vi "Udp Tester 4.vi"() -> ()   [LabVIEW 2014]
uses:
  <vilib>/addons/control/pid/pid.llb/PID (DBL).vi
  <vilib>/addons/control/pid/pid.llb/PID Percentage to EGU (DBL).vi
  <vilib>/FPGAPlugInAG/myRIO-1900/niLvFpga_Open_myRIO-1900.vi
  <vilib>/rvi/interface/common/dynamic/niFpgaDynamicAddResources.vi
  <vilib>/Utility/error.llb/Error Cluster From Error Code.vi
  <vilib>/rvi/errors/niLvFpgaAdjustHostInterfaceError.vi
  <vilib>/FPGAPlugInAG/Dynamic/niLvFpga_Close_Dynamic.vi
  <vilib>/rvi/interface/nirviOpenFPGA/nirviOpenFPGA.xnode
  FPGA Bitfiles/Test_FPGATarget_CurrentControl_60eBuCSPTsI.lvbitx
  Current Control.vi
  <vilib>/rvi/interface/nirviReadWriteControl/nirviReadWriteControl.xnode
  <vilib>/rvi/interface/nirviCloseFPGA/nirviCloseFPGA.xnode
  <vilib>/addons/control/pid/NI_PID_pid.lvlib
  NiFpgaLv.dll
  <vilib>/rvi/interface/Simulation/niFpgaSimulationCallBeginRW.vi
  <vilib>/Utility/file.llb/Write To Spreadsheet File (I64).vi
panel:
  out "Status?":bool
  in  "Tab Control 2":T1(tab)
  out "Plant Output vs. IAB Height":waveform(dbl)[](graph)=[{"t0"=timestamp(1835.8000000000002 s since 1904-01-01), "dt"=1.0, "Y"=[0.9645428084016676]}, {"t0"=timestamp(1835.8000000000002 s since 1904-01-01), "dt"=1.0, "Y"=[1.0]}]
  in  "SP1: 2":dbl(slide)=40.87020302841148 min=0.0 max=0.0 scale=35.0..43.0
  out "Head Pose:":dbl(slide)=50.762476114859936 scale=0.0..100.0
  out "Static Response":cluster{dbl, "Input Signal":dbl}[](graph)
  out "Excitation":cluster{"Time":dbl[], "Signal":dbl[]}(graph)
  out "Response":cluster{"Time":dbl[], "Signal":dbl[]}(graph)
  in  "stop":bool
  out "SP and PV":cluster{"Plant Output":dbl, "SP:":dbl}(graph)
  out "MV (mA)":dbl(graph)=20.39115328927357
  in  "Loop Cycle":i32
  in  "Tab Control":enum32{"Profile", "Diagram"}(tab)
  out "Inflow Profile Graph":cluster{dbl, dbl}[](graph)
  in  "Apply Inflow Profile":bool=TRUE
  in  "Constant Flow (%)":dbl=40.0
  in  "Inflow Profile":cluster{"time (s)":dbl, "setpoint":dbl}[](array[cluster])=[{"time (s)"=0.0, "setpoint"=40.0}, {"time (s)"=10.0, "setpoint"=40.0}, {"time (s)"=10.0, "setpoint"=60.0}, {"time (s)"=20.0, "setpoint"=60.0}]
  out "FT Valve":dbl(knob)=84.28886007445381 scale=0.0..190.0
  out "control valve":dbl=86.66603993277398 format="%.2f"
  out "Valve":bool
  out "Pump":bool=TRUE
  out "Bladder Tank":dbl(slide)=49.279730305904245 scale=0.0..100.0 scale format="%.2f"
  out "FT":dbl(knob)=84.28886007445381 scale=0.0..100.0
  out "PV 1":dbl=49.279730305904245
  in  "Stop":bool
  in  "PID parameters (LC)":T2={"Kc"=-20.0, "Ti (min)"=0.1, "Td (min)"=0.0} {"Td (min)" format="%#.6f"; "Ti (min)" format="%#.4f"; "Kc" format="%#.4f"}
  in  "SP1:":dbl(slide)=40.87020302841148 min=0.0 max=0.0 scale=0.0..100.0
  out "PV1:":dbl(slide)=50.762476114859936 scale=0.0..190.0
  out "MV1:":dbl(slide)=100.0 scale=-100.0..100.0
  # "Time (s)"
  # "Flow (%)"
  # "SP"
  # "///"
  # "///"
  # "///"
  # "1"
  # "///"
  # "SP"
  # "2"
  # "mA"
  # "mA"
  # "FC"
  # "LT"
  # "1"
  # "+"
  # "+"
  # "S"
  # "LC"
  # "FT"
  # "1"
  # "%"
  # "cm"
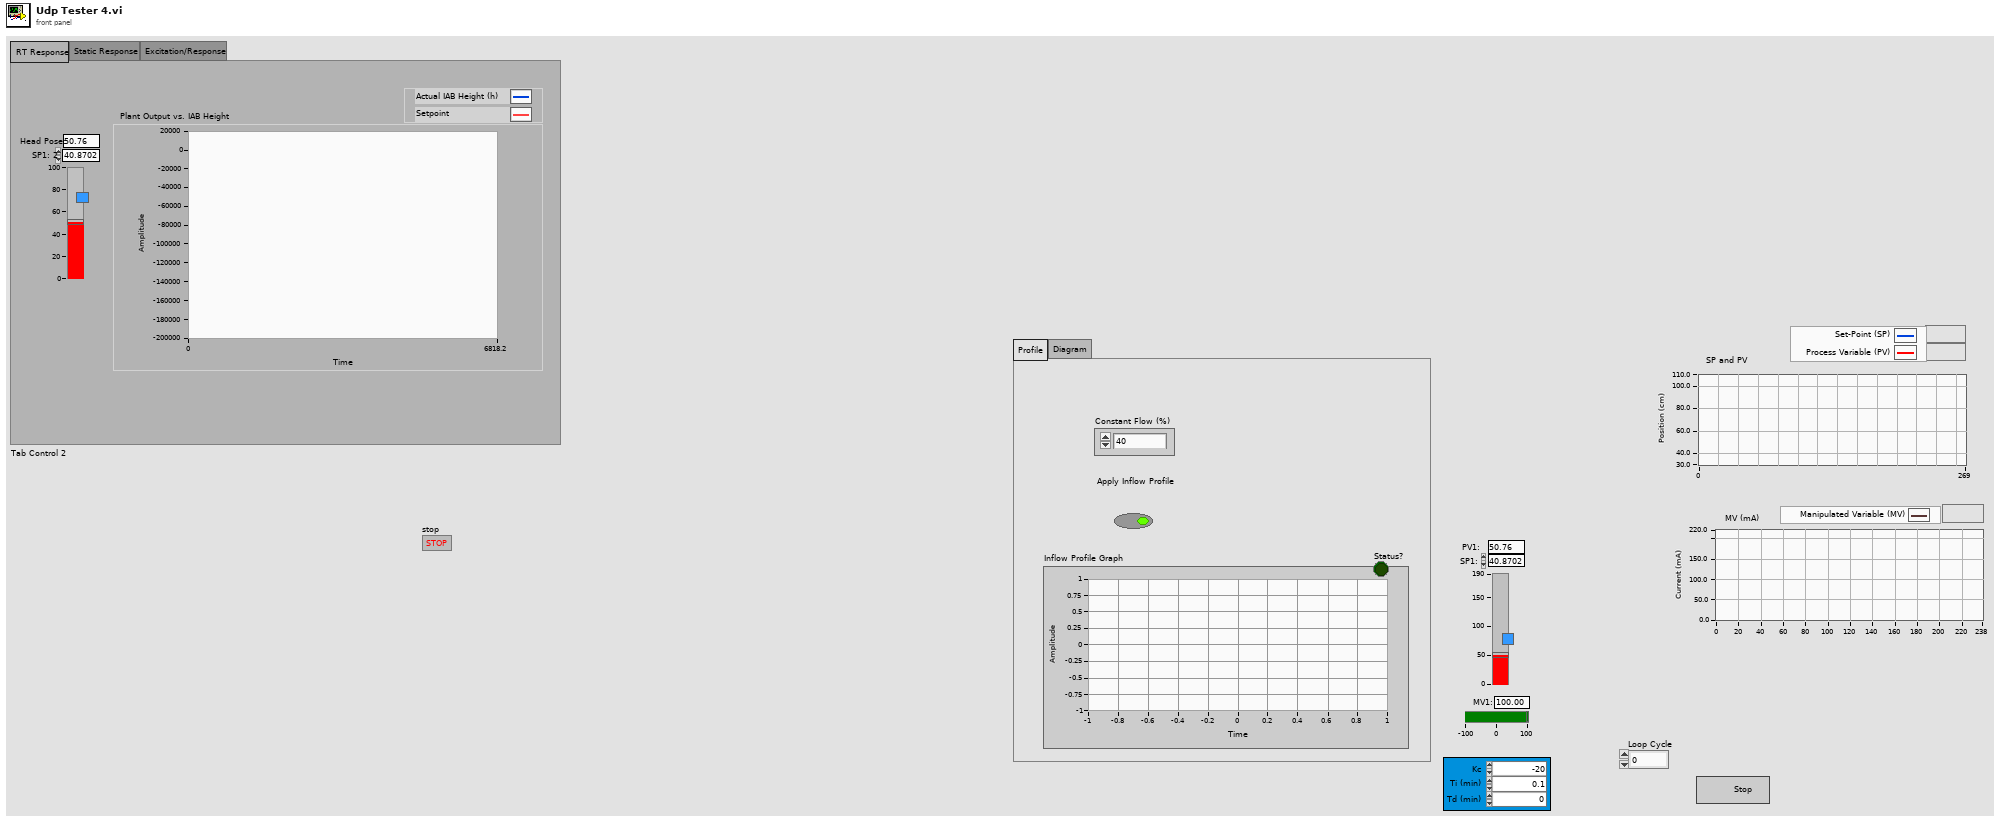
[diagram p1: front panel]
types:
  T1 = enum32{"RT Response", "Static Response", "Excitation/Response"}
  T2 = cluster{"Kc":dbl, "Ti (min)":dbl, "Td (min)":dbl}
  T3 = enum16{"big-endian, network order", "native, host order", "little-endian"}
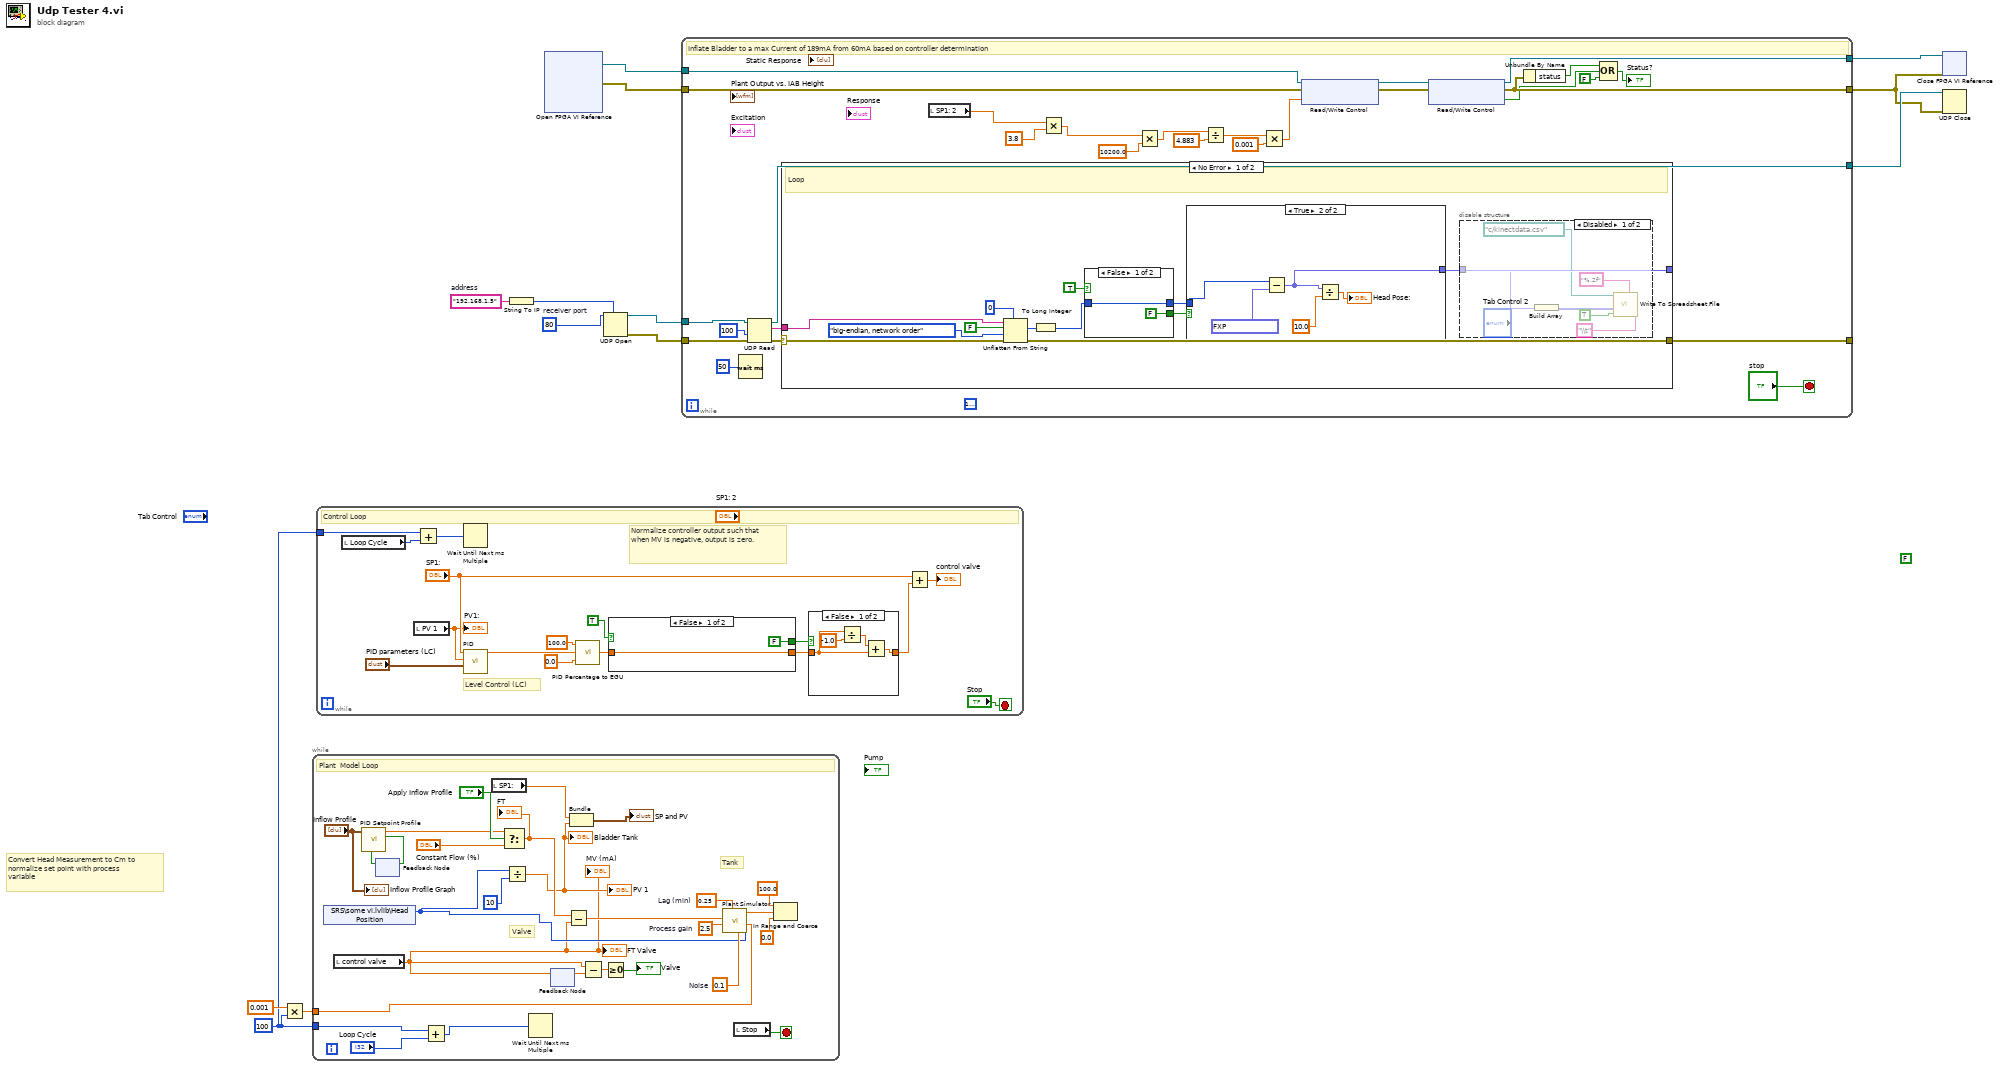
[diagram p0: block diagram]
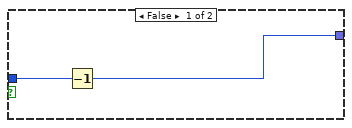
[diagram p3: hidden frame]
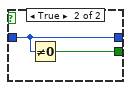
[diagram p4: hidden frame]
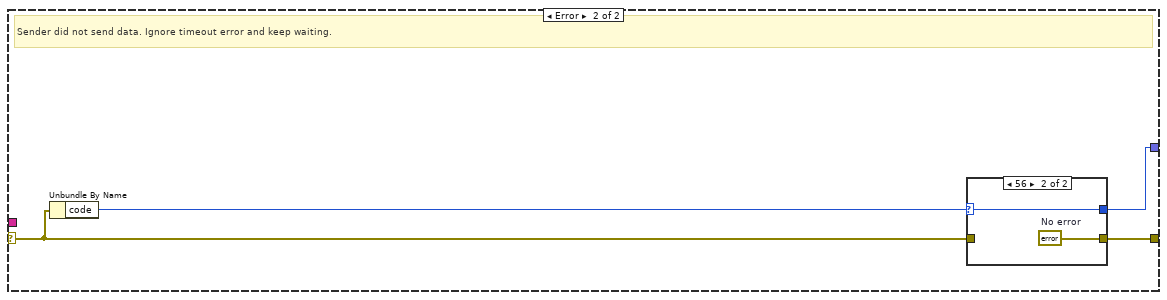
[diagram p5: hidden frame]
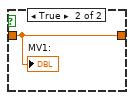
[diagram p7: hidden frame]
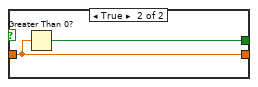
[diagram p8: hidden frame]
diagram:
  w9 = "192.168.1.5"  # address
  w8 = u16 80  # receiver port
  w11 = 100
  (unwired) FALSE
  # "Convert Head Measurement to Cm to normalize set point with process variable"
  n1 = Multiply(x=0.001, y=w11) -> (x*y=w12:dbl)
  n2 = while {
    tunnel: w12 -> [w27]
    tunnel: w11 -> [w18]
    stop <- w39 stop-if-true
    w37 = 0.25  # Lag (min)
    w36 = 2.5  # Process gain
    w35 = 0.1  # Noise
    # "Tank"
    # "Valve"
    # "Plant  Model Loop"
    n3 = shared-variable "SRS\\some vi.lvlib\\Head Position"() -> (w21:i32)  [unwired: 1 in, 1 out]
    n4 = local read "control valve"() -> (w16:dbl)
    "FT Valve" <- w16
    "MV (mA)" <- w16
    n5 = feedback #1() -> (w40:bool)  [unwired: 1 in]
    n6 = call <vilib>:"PID Setpoint Profile.vi"("reinitialize? (F)"=w40, "setpoint profile"="Inflow Profile") -> ("profile complete?"=w41:bool, "setpoint"=w29:dbl)  [unwired: 4 in, 2 out]
    n7 = feedback-in #1(w41) -> ()
    n8 = Add(x=w18, y="Loop Cycle") -> (x+y=w19:i32)
    n9 = local read "SP1:"() -> (w15:dbl)
    n10 = Select(t=w29, s="Apply Inflow Profile", f="Constant Flow (%)") -> (s? t:f=w30:dbl)
    "FT" <- w30
    n11 = Divide(x=w21, y=10 ("x")) -> (x/y=w22:dbl)
    "Bladder Tank" <- w22
    "PV 1" <- w22
    n12 = Wait Until Next ms Multiple(millisecond multiple=w19) -> ()  [unwired: 1 out]
    n13 = feedback-in #2(w16) -> ()
    n14 = feedback #2() -> (w25:dbl)  [unwired: 1 in]
    n15 = Subtract(x=w30, y=w16) -> (x-y=w31:dbl)
    n16 = Bundle("SP1:"=w15, w22) -> (→"SP and PV":cluster{"SP1:":dbl, dbl})  [unwired: 1 in]
    n17 = Subtract(x=w16, y=w25) -> (x-y=w24:dbl)
    n18 = Greater Or Equal To 0?(x=w24) -> (x >= 0?=→"Valve":bool)
    n19 = call "Plant Simulator.vi"("Initial PV"=w21, "dt (s)"=w27, "Controller Noise (%)"=w35, "Lag (min)"=w37, "Process Gain"=w36, "Manipulated Variable (Output, %)"=w31) -> ("Process Variable (%)"=w34:dbl)  [unwired: 5 in]
    n20 = local read "Stop"() -> (w39:bool)
    n21 = In Range and Coerce(upper limit=100.0, x=w34, lower limit=0.0) -> ()  [unwired: 2 out]
    "Inflow Profile Graph" <- "Inflow Profile"
  }
  n22 = while {
    tunnel: w11 -> [w52]
    stop <- "Stop" stop-if-true
    # "Normalize controller output such that when MV is negative, output is zero."
    # "Level Control (LC)"
    # "Control Loop"
    n23 = local read "Loop Cycle"() -> (w51:i32)
    n24 = local read "PV 1"() -> (w54:dbl)
    "PV1:" <- w54
    n25 = Add(x=w52, y=w51) -> (x+y=w50:i32)
    n26 = Wait Until Next ms Multiple(millisecond multiple=w50) -> ()  [unwired: 1 out]
    n27 = call-poly <vilib>:"PID.vi"("PID gains"="PID parameters (LC)", "process variable"=w54, "setpoint"="SP1:") -> ("output"=w45:dbl)  [unwired: 7 in, 1 out]
    n28 = call-poly <vilib>:"PID Percentage to EGU.vi"("minimum (EGU)"=0.0, "% span"=w45, "maximum (EGU)"=100.0) -> ("output (EGU)"=w44:dbl)  [unwired: 1 in]
    n29 = case shown="False" TRUE {
      tunnel: w44 -> [w64 w66]
      tunnel: [FALSE w65] -> w48
      tunnel: [w64 w66] -> w47
      frame False {
      }
      frame True {
        n30 = Greater Than 0?(x=w66) -> (x > 0?=w65:bool)
      }
    }
    n31 = case shown="False" w48 {
      tunnel: w47 -> [w59 w62]
      tunnel: [w58 w62] -> w46
      frame False {
        n32 = Divide(x=w59, y=-1.0) -> (x/y=w61:dbl)
        n33 = Add(x=w61, y=w59) -> (x+y=w58:dbl)
      }
      frame True {
        "MV1:" <- w62
      }
    }
    n34 = Add(x="SP1:", y=w46) -> (x+y=→"control valve":dbl)
  }
  n35 = String To IP(1:w9) -> (0:w10:u32)
  n36 = xnode "Open FPGA VI Reference"() -> ("FPGA VI Reference Out"=w2:refnum<k20>, "error out"=w1:errorcluster)  [unwired: 2 in]
  n37 = UDP Open(7:w10, 11:w8) -> (port=w7:refnum<k16>, 0:w6:errorcluster)  [unwired: 3 in, 1 out]
  n38 = while {
    tunnel: w7 -> [w94]
    tunnel: w6 -> [w93]
    tunnel: w2 -> [w88]
    tunnel: [w89] -> w4
    tunnel: w1 -> [w91]
    tunnel: [w90] -> w3
    tunnel: [w73] -> _
    tunnel: [w72] -> w5
    stop <- "stop" stop-if-true
    (unwired) u32 16777216
    # "Inflate Bladder to a max Current of 189mA from 60mA based on controller determination"
    n39 = Wait (ms)(milliseconds to wait=u32 50) -> ()  [unwired: 1 out]
    n40 = UDP Read(connection ID=w94, timeout ms (25000)=100, 8:w93) -> (data out=w75:string, error out=w74:errorcluster, 3:w72:refnum<k16>)  [unwired: 3 out]
    n41 = case shown="No Error" w74 {
      selector: w74 -> [w101 w126]
      tunnel: w75 -> [w102 _]
      tunnel: [w100 w125] -> w73
      tunnel: [w96 w124] -> _
      frame No Error {
        # "Loop"
        n42 = Unflatten From String(type=0, binary string=w102, data includes array or string size? (T)=FALSE, byte order (0:big-endian, network order)=T3."big-endian, network order" ("byte order"), error in (no error)=w101) -> (value=w103:i32, error out=w100:errorcluster)  [unwired: 1 out]
        n43 = To Long Integer(number=w103) -> (32bit integer=w98:i32)
        n44 = case shown="False" TRUE {
          tunnel: w98 -> [w120 w122]
          tunnel: [FALSE w123] -> w97
          tunnel: [w120 w122] -> w95
          frame False {
          }
          frame True {
            n45 = Not Equal To 0?(x=w122) -> (x != 0?=w123:bool)
          }
        }
        n46 = case shown="True" w97 {
          tunnel: w95 -> [w114 w118]
          tunnel: [w113 w116] -> w96
          frame False {
            n47 = Decrement(x=w114) -> (x-1=w113:i32)
          }
          frame True {
            n48 = Subtract(x=w118, y=fxp<+,18,8> 246.3818359375) -> (x-y=w116:fxp<+/-,43,33>)
            n49 = Divide(x=w116, y=10.0) -> (x/y=→"Head Pose:":dbl)
          }
        }
        n50 = disable-structure shown="Disabled" {
          disable-tunnel: w96 -> [w107 _]
          frame Disabled {
            n51 = Build Array(w107) -> (w112:fxp<+/-,43,33>[])
            n52 = call-poly <vilib>:"Write To Spreadsheet File.vi"("delimiter (\\t)"="\\t" ("delimiter (\\t)"), "format (%d)"="%.2f", "append to file? (new file:F)"=TRUE, "1D data"=w112, "file path (dialog if empty)"=path "c:/kinectdata.csv") -> ()  [unwired: 3 in, 1 out]
          }
          frame Enabled {
          }
        }
      }
      frame Error {
        # "Sender did not send data. Ignore timeout error and keep waiting."
        n53 = Unbundle By Name(w126) -> ("code"=w127:i32)
        n54 = case shown="56" w127 {
          selector: w127 -> [w128 w130]
          tunnel: w126 -> [w129 _]
          tunnel: [w129 w131] -> w125
          tunnel: [w128 w130] -> w124
          frame Default {
          }
          frame 56 {
            w131 = errorcluster {"status"=FALSE, "code"=0, "source"=""}  # No error
          }
        }
      }
    }
    n55 = local read "SP1: 2"() -> (w67:dbl)
    n56 = Multiply(x=w67, y=3.8) -> (x*y=w69:dbl)
    n57 = Multiply(x=w69, y=10200.0) -> (x*y=w76:dbl)
    n58 = Divide(x=w76, y=4.883) -> (x/y=w79:dbl)
    n59 = Multiply(x=w79, y=0.001) -> (x*y=w85:dbl)
    n60 = xnode "Read/Write Control"("FPGA VI Reference In"=w88, "error in"=w91, "DAC Inlet Valve"=w85) -> ("FPGA VI Reference Out"=w87:refnum<k20>, "error out"=w86:errorcluster)
    n61 = xnode "Read/Write Control"("FPGA VI Reference In"=w87, "error in"=w86) -> ("FPGA VI Reference Out"=w89:refnum<k20>, "error out"=w90:errorcluster, "Inlet Overflow?"=w84:bool)
    n62 = Unbundle By Name(w90) -> ("status"=w82:bool)
    n63 = Compound Arithmetic op=OR(w82, w84, FALSE ("value")) -> (→"Status?":bool)
  }
  n64 = xnode "Close FPGA VI Reference"("FPGA VI Reference In"=w4, "error in"=w3) -> ()  [unwired: 1 out]
  n65 = UDP Close(connection ID=w5, 8:w3) -> ()  [unwired: 2 out]
